vi "MarvinTester.vi"() -> ()   [LabVIEW 2017]
uses:
  <vilib>/Instr/_visa.llb/VISA Configure Serial Port (Instr).vi
panel:
  out "TX":string
  out "RX":string
  out "(hi.lo)":u32 format="%.0x"
  in  "GetOUTIO3":bool
  out "S2 GIO 19":bool
  out "S2 GIO 18":bool
  out "S2 GIO 17":bool
  out "S2 GIO 11":bool
  out "S2 GIO 3":bool
  out "S2 GIO 1":bool
  out "S1 GIO 19":bool
  out "S1 GIO 18":bool
  out "S1 GIO 17":bool
  out "S1 GIO 15":bool
  out "S1 GIO 11":bool
  out "S1 GIO 3":bool
  out "S1 GIO 1":bool
  in  "GetIO 2":bool
  out "S2 GIO 15 R":bool
  in  "Reset":bool
  in  "SetDefault":bool
  out "GetIO":u8[](array[numeric])
  out "Ver":string=" "
  in  "Get  ver":bool
  out "PWM Reading":u32
  out "Time Plot":i32=-1
  out "error out":errorcluster
  in  "stop":bool
  in  "Ring":u16(ring) items=["None", "Moment", "Get IO"]
  out "packet PWM":u8[](array[numeric])
  in  "Tab Control":enum32{"Page 3", "Page 4", "Page 2"}(tab)
  in  "GetIO2":bool
  out "out_io1":u32 format="%.0b"
  in  "SetDAC":bool
  in  "I_O":u32 format="%.0b"
  in  "ADC":bool
  in  "ADC num":u8=3
  out "out_io1 2":u32
  in  "DAC":u32
  in  "idx":i32
  in  "TA[idx]":bool
  in  "Disconect 2":bool
  in  "110":bool
  in  "120":bool
  in  "90":bool
  in  "60":bool
  in  "100":bool
  in  "20":bool
  in  "70":bool
  in  "40":bool
  in  "30":bool
  in  "80":bool
  in  "50":bool
  in  "10":bool
  in  "25":bool
  in  "0":bool
  in  "COM Port Marvin":refnum<visa-resource-name>="COM1"
  in  "Connect Marvin":bool
  out "CommIcon Marvin":bool=TRUE
  out "String":string
  in  "K15":bool
  in  "Firmeware":bool
  in  "K16":bool
  in  "K17":bool
  in  "Power":bool
  in  "Fan":bool
  in  "VEnable":bool
  out "CurrSp Graph":cluster{"n":dbl, "T":dbl}[](graph)
  out "Frequency":dbl
  in  "Plot On":bool
  in  "Plot OFF":bool
  in  "Get":bool
  in  "Clear":bool
  in  "Plot Time":i32=70
  out "Load":dbl
  out "String 2":string
  in  "COM Port Control":refnum<visa-resource-name>="COM1"
  in  "Time":i32=-1
  out "err tx":errorcluster
  out "Write array":u8[](array[numeric]) format="%x"
  in  "Flag Stop T":bool
  out "VISA":refnum<visa-resource-name>
  out "CommIcon":bool=TRUE
  out "Read array":u8[](array[numeric]) format="%x"
  out "Cmd Id":u8
  in  "Flag Stop I":bool=TRUE
  out "Int b":i32
  in  "Flag Stop R":bool
  out "TX":bool
  out "RX":bool
  in  "Command Menu 2":u16(ring) items=["Status", "Moment", "Isc threshold", "Vin Vout", "RESET FF", "Open", "Close", "Up Time", "Interval Period", "Nm Of Retries", "On time", "Save Parameters", "Version", "Temperature"]
  out "packet":u8[](array[numeric])
  in  "Isc1":i8
  in  "Add Unit":u8
  in  "Disconect":bool
  in  "Connect":bool
  in  "Stop VI":bool
  out "status":bool
  # "Marvin Tester"
  # "[Hz]"
  # "SW Version"
  # "ver : 00.01.b"
  # "I/O"
  # "ADC"
  # "DAC"
  # "0-4"
  # "V=ADC*3.3/4096"
  # "Term1  -0\nTerm2  -1\nCurr   - 2\nEBAYFAN -3\nTempCPU -4"
  # "b0-Rly1\nb1-Rly2\nb2-Rly3\n....\nb20-Rly20\nb21-Power"
  # "[kHz]"
  # "[N.m]"
  # "[msec]"
  # "ver 0.0.1"
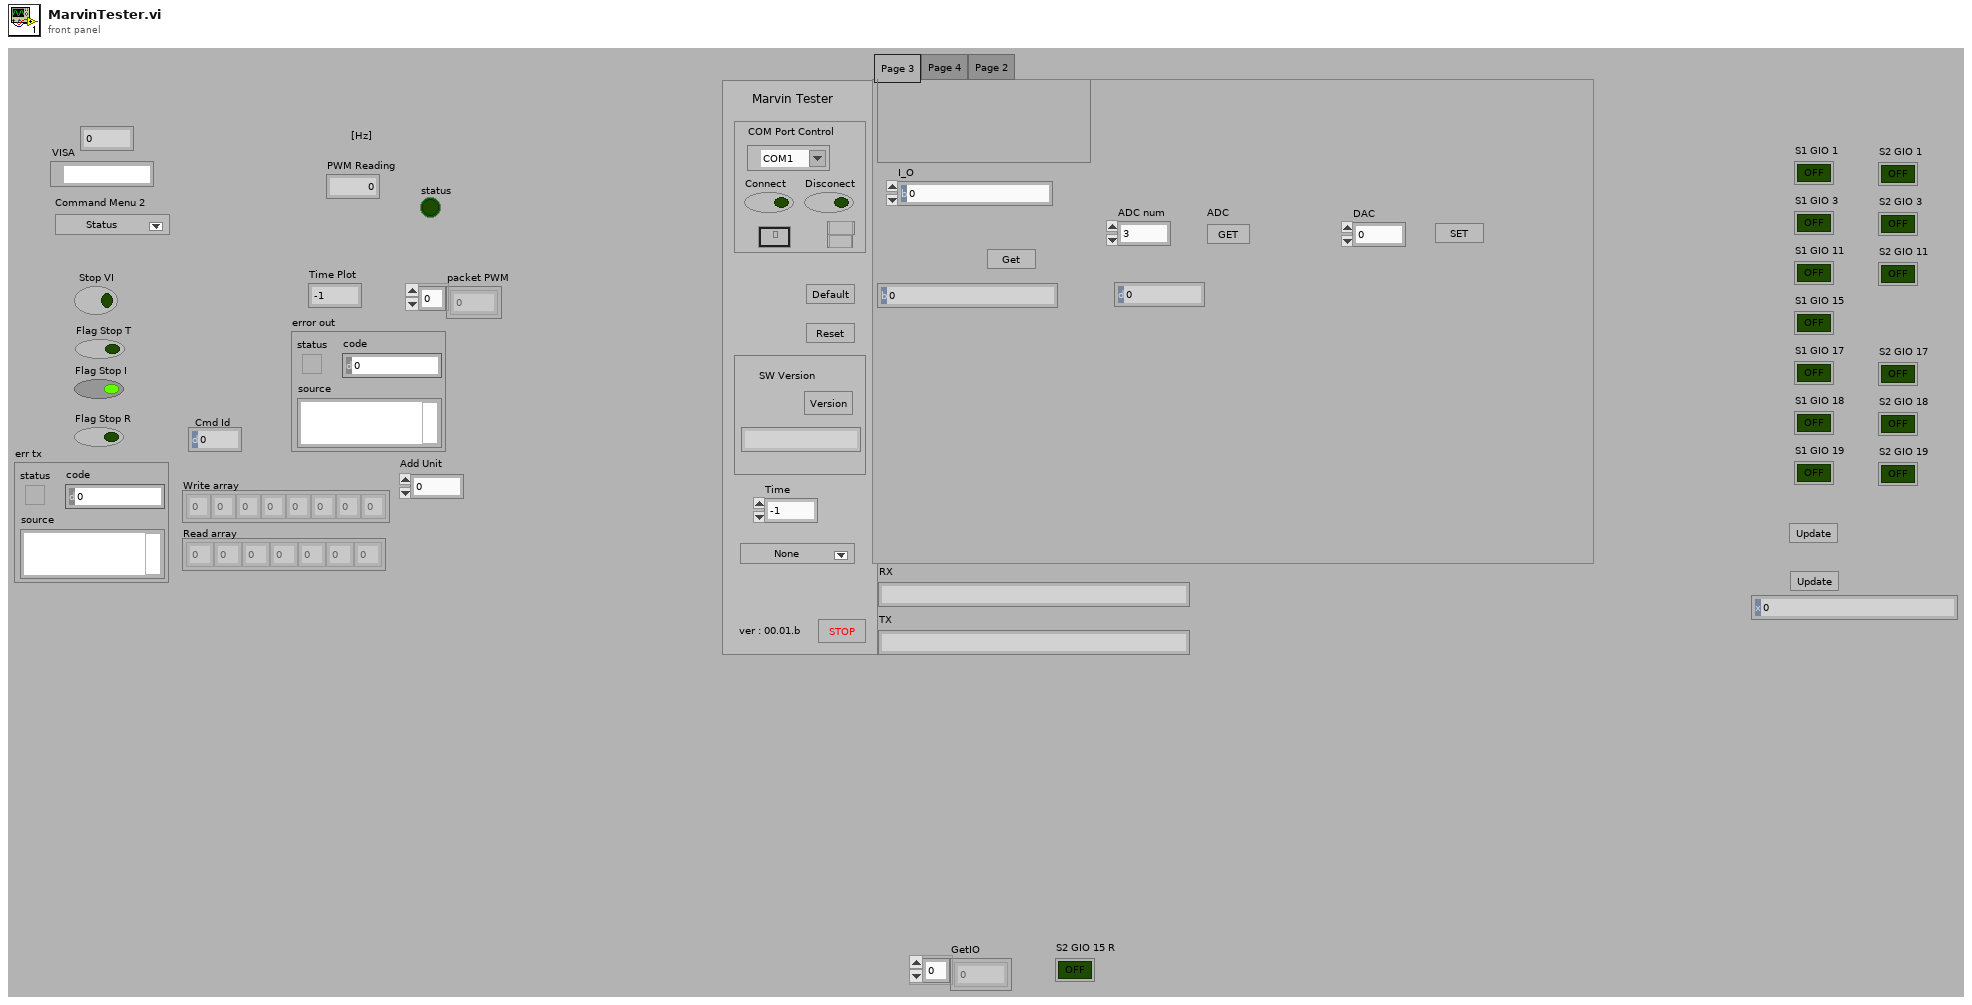
[diagram p1: front panel]
types:
  T1 = cluster{"d1":dbl, "d2":dbl, "d3":dbl, "id":u16, "d4":dbl}
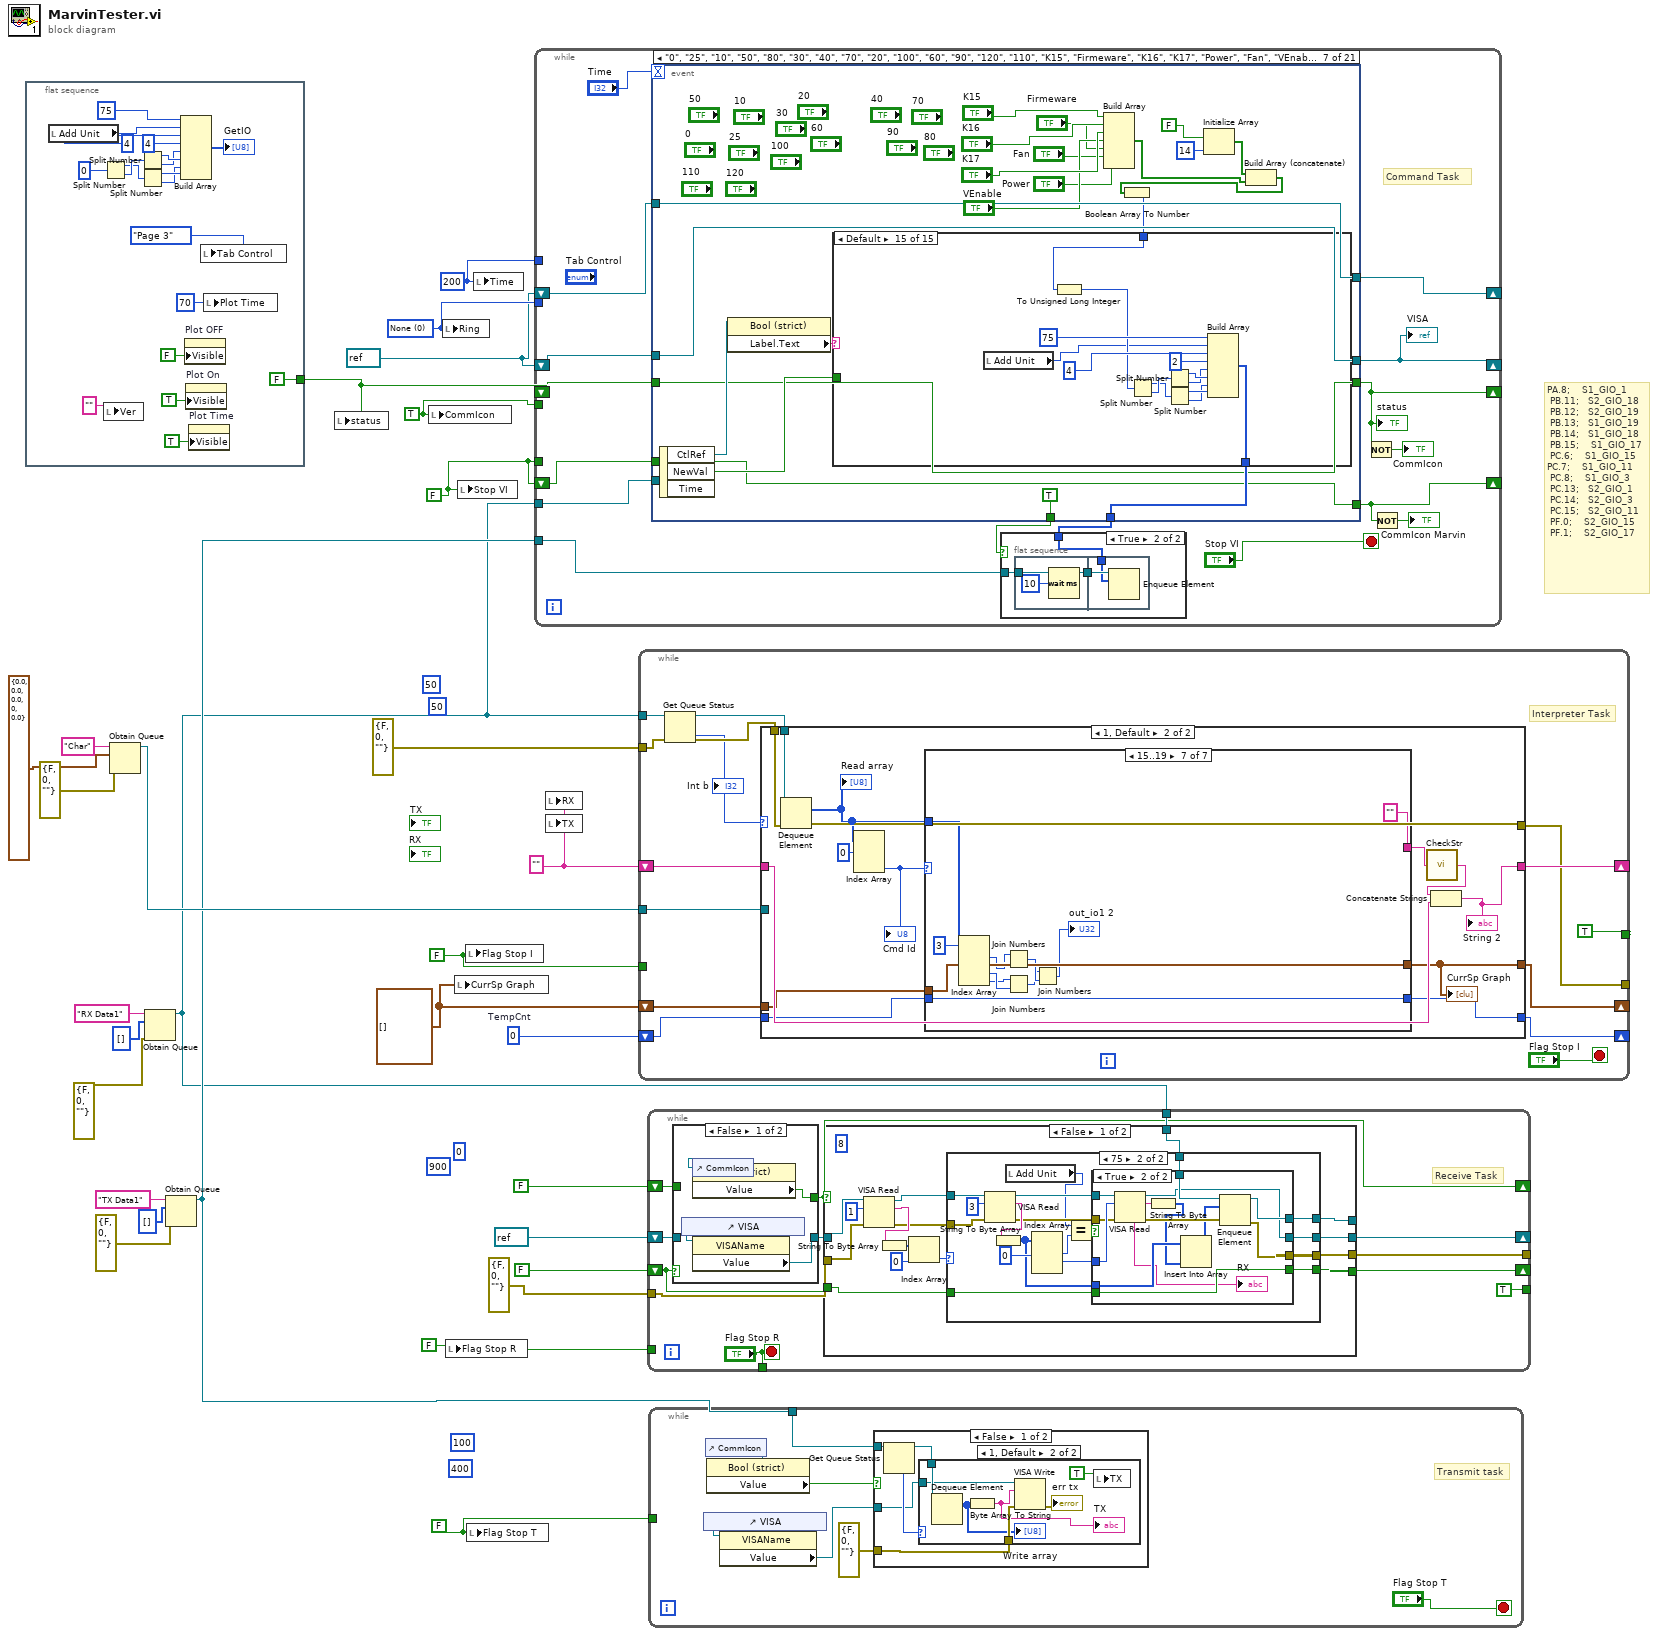
[diagram p0: block diagram]
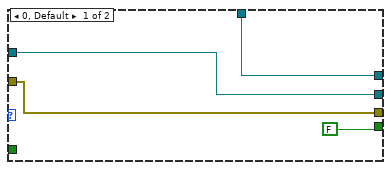
[diagram p3: hidden frame]
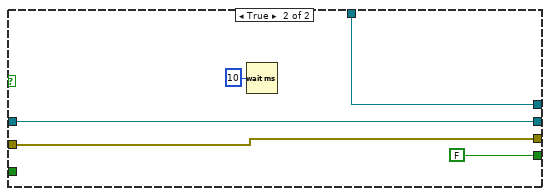
[diagram p5: hidden frame]
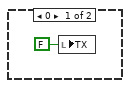
[diagram p6: hidden frame]
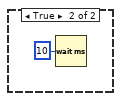
[diagram p7: hidden frame]
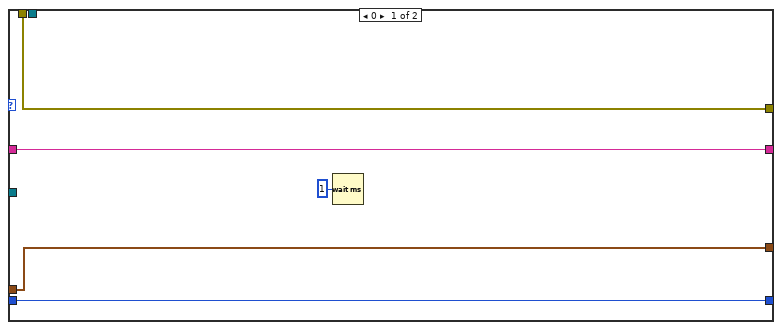
[diagram p8: hidden frame]
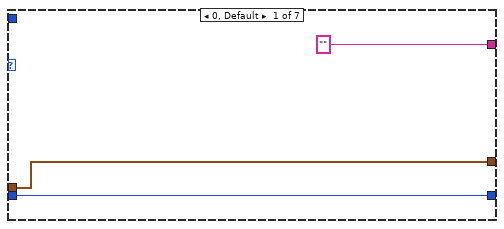
[diagram p9: hidden frame]
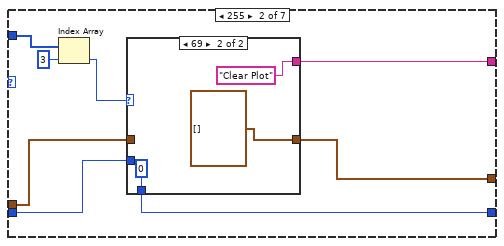
[diagram p10: hidden frame]
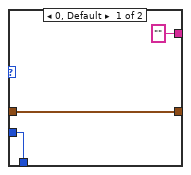
[diagram p11: hidden frame]
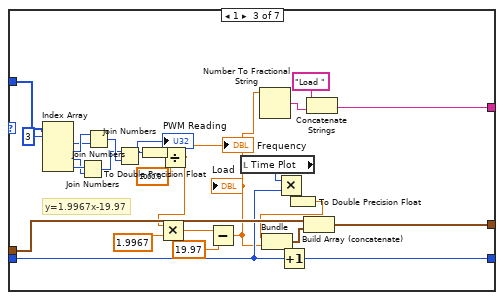
[diagram p12: hidden frame]
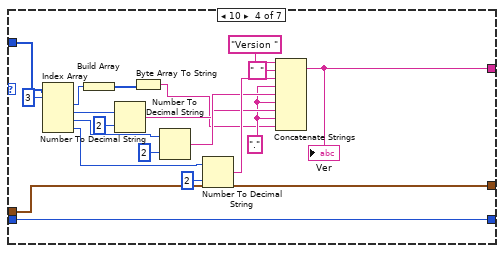
[diagram p13: hidden frame]
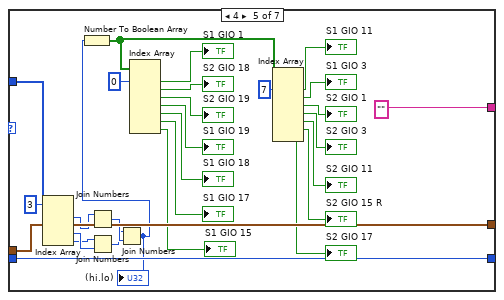
[diagram p14: hidden frame]
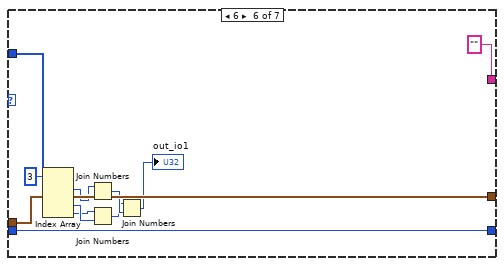
[diagram p15: hidden frame]
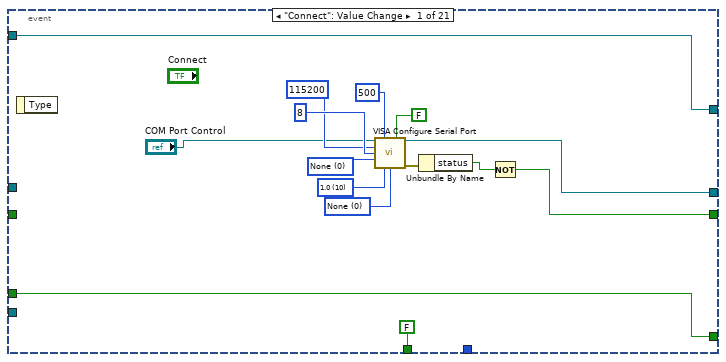
[diagram p17: hidden frame]
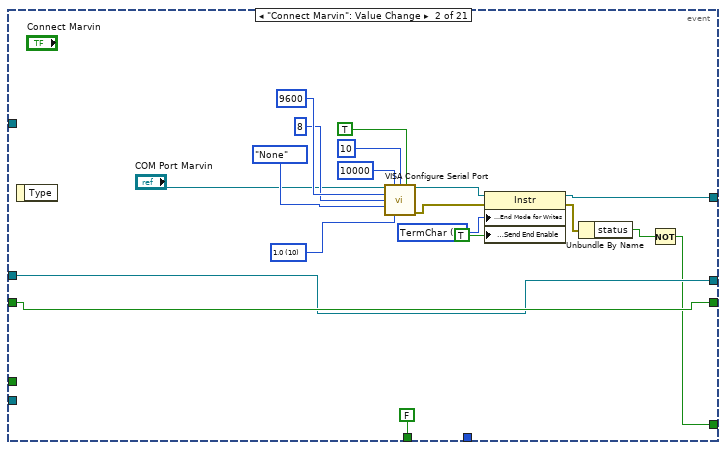
[diagram p18: hidden frame]
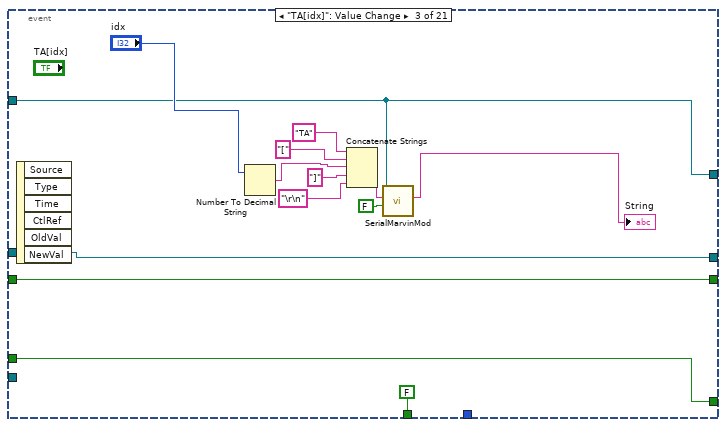
[diagram p19: hidden frame]
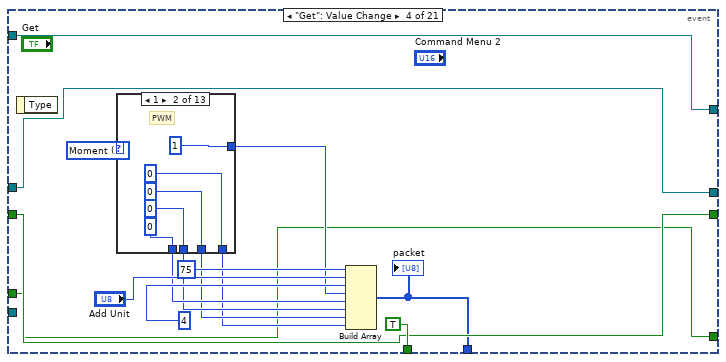
[diagram p20: hidden frame]
diagram:
  w8 = u16 0  # TempCnt
  w5 = cluster{"n":dbl, "T":dbl}[] [] ("Current Graph 4")
  w9 = 200 ("Time")
  w10 = u16 0 items=["None", "Moment"] ("Ring")
  w11 = TRUE ("CommIcon")
  w2 = FALSE
  (unwired) 400 ("Priority")
  (unwired) i64 100 ("Period")
  (unwired) i64 50 ("Period")
  (unwired) 50 ("Priority")
  (unwired) 900 ("Priority")
  (unwired) i64 0 ("Period")
  w14 = FALSE
  w1 = ""
  w28 = FALSE
  w29 = FALSE
  w3 = refnum<visa-resource-name> refnum ("VISA resource name out")
  # "PA.8;   \tS1_GIO_1\n\tPB.11;  \tS2_GIO_18\n\tPB.12;  \tS2_GIO_19\n\tPB.13;  \tS1_GIO_19\n\tPB.14;  \tS1_GIO_18\n\tPB.15;   \tS1_GIO_17\n\tPC.6;   \tS1_GIO_15\nPC.7;   \tS1_GIO_11\n\tPC.8;   \tS1_GIO_3\n\tPC.13;  \tS2_GIO_1\n\tPC.14;  \tS2_GIO_3\n\tPC.15;  \tS2_GIO_11\n\tPF.0;  \t\tS2_GIO_15\n\tPF.1;  \t\tS2_GIO_17"
  n1 = flat-sequence {
    tunnel: [FALSE] -> w7
    frame #0 {
      n2 = local read "Add Unit"() -> (w39:u8)
      n3 = Split Number(x=u32 0) -> (hi(x)=w37:u16, lo(x)=w38:u16)
      n4 = local write "Ver"("" ("Ver")) -> ()
      n5 = Split Number(x=w38) -> (hi(x)=w36:u8, lo(x)=w35:u8)
      n6 = Split Number(x=w37) -> (hi(x)=w34:u8, lo(x)=w33:u8)
      n7 = Build Array(u8 75, w39, u8 4 ("Length"), u8 4, w35, w36, w33, w34) -> (→"GetIO":u8[])
      n8 = property on="Plot OFF" class="Bool"("Visible"=FALSE) -> ()  [unwired: 2 in, 2 out]
      n9 = property on="Plot On" class="Bool"("Visible"=TRUE) -> ()  [unwired: 2 in, 2 out]
      n10 = property on="Plot Time" class="DigNum (strict)"("Visible"=TRUE) -> ()  [unwired: 2 in, 2 out]
      n11 = local write "Tab Control"(enum32{"Page 3", "Page 4", "Page 2"}."Page 3" ("Tab Control")) -> ()
      n12 = local write "Plot Time"(70 ("Plot Time")) -> ()
    }
  }
  n13 = Obtain Queue(name (unnamed)="Char", element data type=T1 {"d1"=0.0, "d2"=0.0, "d3"=0.0, "id"=0, "d4"=0.0}, error in (no error)=errorcluster {"status"=FALSE, "code"=0, "source"=""}) -> (queue out=w19:refnum<queue>)  [unwired: 2 in, 2 out]
  n14 = Obtain Queue(name (unnamed)="RX Data1", element data type=u8[] [], error in (no error)=errorcluster {"status"=FALSE, "code"=0, "source"=""}) -> (queue out=w6:refnum<queue>)  [unwired: 2 in, 2 out]
  n15 = Obtain Queue(name (unnamed)="TX Data1", element data type=u8[] [], error in (no error)=errorcluster {"status"=FALSE, "code"=0, "source"=""}) -> (queue out=w13:refnum<queue>)  [unwired: 2 in, 2 out]
  n16 = local write "status"(w7) -> ()
  n17 = local write "CommIcon"(w11) -> ()
  n18 = local write "Ring"(w10) -> ()
  n19 = local write "Flag Stop R"(w29) -> ()
  n20 = local write "CurrSp Graph"(w5) -> ()
  n21 = local write "Stop VI"(w2) -> ()
  n22 = local write "Flag Stop I"(w28) -> ()
  n23 = local write "Flag Stop T"(w14) -> ()
  n24 = local write "Time"(w9) -> ()
  n25 = while {
    shift-right: [w57] -> _
    shift-left: w3 -> [w64]
    shift-right: [w56] -> _
    shift-left: w7 -> [w63]
    tunnel: w13 -> [w59]
    tunnel: w2 -> [_]
    tunnel: w11 -> [_]
    tunnel: w10 -> [_]
    tunnel: w9 -> [_]
    tunnel: w6 -> [w54]
    shift-right: [w52] -> _
    shift-left: w3 -> [w51]
    shift-right: [w50] -> _
    shift-left: w2 -> [w49]
    stop <- "Stop VI" stop-if-true
    # "Command Task"
    n26 = event shown="[6] \"0\", \"25\", \"10\", \"50\", \"80\", \"30\", \"40\", \"70\", \"20\", \"100\", \"60\", \"90\", \"120\", \"110\", \"K15\", \"Firmeware\", \"K16\", \"K17\", \"Power\", \"Fan\", \"VEnable\": Value Change" {
      selector: _ -> [_ _ _ _ _ _ _ _ _ _ _ _ _ _ _ _ _ _ _ _ _]
      dyn-events: _ -> [_ _ _ _ _ _ _ _ _ _ _ _ _ _ _ _ _ _ _ _ _]
      timeout: "Time" -> [_ _ _ _ _ _ _ _ _ _ _ _ _ _ _ _ _ _ _ _ _]
      tunnel: [w80 w103 w109 w124 w206 w284 w315 w568 w579 w596 w613 w630 w647 w664 w693 w703 w710 w714 refnum<visa-resource-name> refnum ("VISA resource name out") w729 w738] -> w57
      tunnel: w64 -> [_ w103 w109 w124 w206 w284 w315 w568 w579 w596 w613 w630 w647 w664 w693 w703 w710 w714 w725 w729 w738]
      tunnel: [w78 w104 w108 w123 w205 w294 w314 w571 w587 w604 w621 w638 w655 w672 w695 w705 w712 FALSE FALSE w727 w737] -> w56
      tunnel: w63 -> [_ w104 w108 w123 w205 w294 w314 w571 w587 w604 w621 w638 w655 w672 w695 w705 w712 _ _ w727 w737]
      tunnel: [_ _ _ w122 w204 w293 w317 w570 w577 w594 w611 w628 w645 w662 _ _ _ _ _ _ w735] -> w58
      tunnel: [FALSE FALSE FALSE TRUE TRUE TRUE TRUE TRUE TRUE TRUE TRUE TRUE TRUE TRUE FALSE FALSE FALSE FALSE FALSE FALSE w736] -> w60
      tunnel: w54 -> [_ _ _ _ _ _ _ _ _ _ _ _ _ _ _ _ w709 _ _ _ _]
      tunnel: [w73 w90 w110 w121 w201 w282 w313 w563 w576 w593 w610 w627 w644 w661 w678 w697 w707 w715 w721 refnum<visa-resource-name> refnum ("VISA resource name out") w733] -> w52
      tunnel: w51 -> [w73 _ w110 w121 w201 w282 w313 w563 w576 w593 w610 w627 w644 w661 w678 w697 w707 w715 w721 w728 w733]
      tunnel: [w72 w87 w106 w120 w200 w281 w312 w562 w575 w592 w609 w626 w643 w660 w677 w696 w706 w713 w720 FALSE w732] -> w50
      tunnel: w49 -> [w72 _ w106 w120 w200 w281 w312 w562 w575 w592 w609 w626 w643 w660 w677 w696 w706 w713 w720 _ w732]
      event "Connect": Value Change {
        w86 = u16 0 items=["None"=0, "XON/XOFF"=1, "RTS/CTS"=2, "DTR/DSR"=4] ("flow control")
        w85 = u16 10 items=["1.0"=10, "1.5"=15, "2.0"=20] ("stop bits")
        w84 = u16 0 items=["None", "Odd", "Even", "Mark", "Space"] ("parity")
        n27 = event-data() -> ()  [unwired: 1 in, 1 out]
        n28 = call-poly "VISA Configure Serial Port"("VISA resource name"="COM Port Control", "timeout (10sec)"=u32 500, "Enable Termination\nChar (T)"=FALSE ("Enable Termination\nChar (T)"), "baud rate (9600)"=u32 115200 ("baud rate"), "data bits (8)"=u16 8 ("data bits"), "parity (0:none)"=w84, "stop bits (10: 1 bit)"=w85, "flow control (0:none)"=w86) -> ("VISA resource name out"=w80:refnum<visa-resource-name>, "error out"=w77:errorcluster)  [unwired: 6 in]
        n29 = Unbundle By Name(w77) -> ("status"=w79:bool)
        n30 = Not(x=w79) -> (.not. x?=w78:bool)
      }
      event "Connect Marvin": Value Change {
        w102 = u16 2 items=["None", "LastBit", "TermChar", "Break"] ("Serial Settings:Serial End Mode for Writes")
        w95 = u16 10 items=["1.0"=10, "1.5"=15, "2.0"=20] ("stop bits (10: 1 bit)")
        n31 = event-data() -> ()  [unwired: 1 in, 1 out]
        n32 = call-poly "VISA Configure Serial Port"("VISA resource name"="COM Port Marvin", "timeout (10sec)"=u32 10000, "termination char\n(0xA = '\\n' = LF)"=u8 10 ("termination char\n(0xA = '\\n' = LF)"), "Enable Termination\nChar (T)"=TRUE ("Enable Termination\nChar (T)"), "baud rate (9600)"=u32 9600, "data bits (8)"=u16 8, "parity (0:none)"=enum16{"None", "Odd", "Even", "Mark", "Space"}."None", "stop bits (10: 1 bit)"=w95) -> ("VISA resource name out"=w93:refnum<visa-resource-name>, "error out"=w92:errorcluster)  [unwired: 6 in]
        n33 = property class="Instr"(reference=w93, error in=w92, "Serial Settings:End Mode for Writes"=w102, "Message Based Settings:Send End Enable"=TRUE) -> (reference out=w90:refnum<visa-resource-name>, error out=w88:errorcluster)
        n34 = Unbundle By Name(w88) -> ("status"=w89:bool)
        n35 = Not(x=w89) -> (.not. x?=w87:bool)
      }
      event "TA[idx]": Value Change {
        n36 = event-data() -> ()  [unwired: 1 in, 6 out]
        n37 = Number To Decimal String(number="idx") -> (decimal integer string=w113:string)  [unwired: 1 in]
        n38 = Concatenate Strings("TA" ("string"), "[", w113, "]", "\r\n" ("write buffer")) -> (w114:string)
        n39 = call "SerialMarvinMod.vi"("Clear Log"=FALSE, "write buffer"=w114, "VISA resource name"=w110) -> ("read buffer"=→"String":string)  [unwired: 7 in, 1 out]
      }
      event "Get": Value Change {
        w126 = u16 1 items=["Status", "Moment", "Isc threshold", "Vin Vout", "RESET FF", "Open", "Close", "Up Time", "Interval Period", "Nm Of Retries", "On time", "Save Parameters", "Version", "Temperature"] ("Command Menu 3")
        n40 = event-data() -> ()  [unwired: 1 in, 1 out]
        n41 = case shown="1" w126 {
          tunnel: [u8 0 u8 1 u8 2 u8 15 u8 4 u8 4 u8 5 u8 6 u8 7 u8 8 u8 9 u8 10 u8 16] -> w131
          tunnel: [u8 0 u8 0 u8 0 u8 0 u8 0 u8 0 u8 0 u8 0 u8 0 u8 0 u8 0 u8 0 u8 0] -> w129
          tunnel: [u8 0 u8 0 u8 0 u8 0 u8 0 u8 0 u8 0 u8 0 u8 0 u8 0 u8 0 u8 0 u8 0] -> w128
          tunnel: [u8 0 u8 0 "Isc1" u8 0 u8 1 u8 0 u8 0 u8 0 u8 0 u8 0 u8 0 u8 0 u8 0] -> w130
          tunnel: [u8 0 u8 0 u8 0 u8 0 u8 0 u8 0 u8 0 u8 0 u8 0 u8 0 u8 0 u8 0 u8 0] -> w127
          frame 0, Default {
            # "Status"
          }
          frame 1 {
            # "PWM"
          }
          frame 2 {
          }
          frame 3 {
            # "Vout"
          }
          frame 5 {
          }
          frame 6 {
          }
          frame 7 {
          }
          frame 8 {
          }
          frame 9 {
          }
          frame 10 {
          }
          frame 11 {
          }
          frame 12 {
          }
          frame 13 {
          }
        }
        n42 = Build Array(u8 75, "Add Unit", u8 4 ("Length"), w131, w130, w129, w128, w127) -> (w122:u8[])
        "packet" <- w122
      }
      event "Get  ver": Value Change {
        w208 = u16 12 items=["Status", "Moment", "Isc threshold", "Vin Vout", "RESET FF", "Open", "Close", "Up Time", "Interval Period", "Nm Of Retries", "On time", "Save Parameters", "Version", "Temperature"] ("Command Menu 3")
        n43 = event-data() -> ()  [unwired: 1 in, 1 out]
        n44 = local read "Add Unit"() -> (w203:u8)
        n45 = case shown="0, Default" w208 {
          tunnel: [u8 0 u8 1 u8 2 u8 15 u8 4 u8 4 u8 5 u8 6 u8 7 u8 8 u8 9 u8 10 u8 16] -> w213
          tunnel: [u8 0 u8 0 u8 0 u8 0 u8 0 u8 0 u8 0 u8 0 u8 0 u8 0 u8 0 u8 0 u8 0] -> w211
          tunnel: [u8 0 u8 0 u8 0 u8 0 u8 0 u8 0 u8 0 u8 0 u8 0 u8 0 u8 0 u8 0 u8 0] -> w210
          tunnel: [u8 0 u8 0 u8 0 u8 0 u8 1 u8 0 u8 0 u8 0 u8 0 u8 0 u8 0 u8 0 u8 0] -> w212
          tunnel: [u8 0 u8 0 u8 0 u8 0 u8 0 u8 0 u8 0 u8 0 u8 0 u8 0 u8 0 u8 0 u8 0] -> w209
          frame 0, Default {
            # "Status"
          }
          frame 1 {
            # "PWM"
          }
          frame 2 {
          }
          frame 3 {
            # "Vout"
          }
          frame 5 {
          }
          frame 6 {
          }
          frame 7 {
          }
          frame 8 {
          }
          frame 9 {
          }
          frame 10 {
          }
          frame 11 {
          }
          frame 12 {
          }
          frame 13 {
          }
        }
        n46 = local write "Ver"("" ("Ver")) -> ()
        n47 = Build Array(u8 75, w203, u8 4 ("Length"), w213, w212, w211, w210, w209) -> (w204:u8[])
      }
      event "I_O": Value Change {
        n48 = event-data() -> ()  [unwired: 1 in, 3 out]
        n49 = local read "Add Unit"() -> (w292:u8)
        n50 = To Unsigned Long Integer(number="I_O") -> (unsigned 32bit integer=w285:u32)
        n51 = Split Number(x=w285) -> (hi(x)=w290:u16, lo(x)=w291:u16)
        n52 = Split Number(x=w291) -> (hi(x)=w289:u8, lo(x)=w288:u8)
        n53 = Split Number(x=w290) -> (hi(x)=w287:u8, lo(x)=w286:u8)
        n54 = Build Array(u8 75, w292, u8 4 ("Length"), u8 2, w288, w289, w286, w287) -> (w293:u8[])
      }
      event "0", "25", "10", "50", "80", "30", "40", "70", "20", "100", "60", "90", "120", "110", "K15", "Firmeware", "K16", "K17", "Power", "Fan", "VEnable": Value Change {
        n55 = event-data() -> ("CtlRef"=w320:refnum<vi>, "NewVal"=w318:bool)  [unwired: 1 in, 1 out]
        n56 = property class="Bool (strict)"(reference=w320) -> ("Label.Text"=w319:string)  [unwired: 1 in, 2 out]
        n57 = Build Array("K15", "K16", "K17", "VEnable", "Firmeware", "Fan", "Power") -> (w300:bool[])
        n58 = Initialize Array(FALSE, 14 ("dimension size")) -> (w301:bool[])
        n59 = Build Array (concatenate)(w301, w300) -> (w299:bool[])
        n60 = Boolean Array To Number(Boolean array=w299) -> (number=w304:u32)
        n61 = case shown="Default" w319 {
          tunnel: w318 -> [w325 w341 w356 w372 w388 w404 w420 w436 w455 w470 w489 w504 w520 w536 _]
          tunnel: [w322 w338 w353 w369 w385 w401 w417 w433 w452 w467 w486 w501 w517 w533 w549] -> w317
          tunnel: w304 -> [_ _ _ _ _ _ _ _ w451 _ w484 _ _ _ w550]
          frame "0" {
            n62 = Select(t=u32 1 ("number"), s=w325, f=u32 0) -> (s? t:f=w323:u32)
            n63 = local read "Add Unit"() -> (w326:u8)
            n64 = To Unsigned Long Integer(number=w323) -> (unsigned 32bit integer=w327:u32)
            n65 = Split Number(x=w327) -> (hi(x)=w332:u16, lo(x)=w333:u16)
            n66 = Split Number(x=w333) -> (hi(x)=w331:u8, lo(x)=w330:u8)
            n67 = Split Number(x=w332) -> (hi(x)=w329:u8, lo(x)=w328:u8)
            n68 = Build Array(u8 75, w326, u8 4 ("Length"), u8 2, w330, w331, w328, w329) -> (w322:u8[])
          }
          frame "10" {
            n69 = Select(t=u32 2 ("number"), s=w341, f=u32 0) -> (s? t:f=w339:u32)
            n70 = local read "Add Unit"() -> (w342:u8)
            n71 = To Unsigned Long Integer(number=w339) -> (unsigned 32bit integer=w343:u32)
            n72 = Split Number(x=w343) -> (hi(x)=w348:u16, lo(x)=w349:u16)
            n73 = Split Number(x=w349) -> (hi(x)=w347:u8, lo(x)=w346:u8)
            n74 = Split Number(x=w348) -> (hi(x)=w345:u8, lo(x)=w344:u8)
            n75 = Build Array(u8 75, w342, u8 4 ("Length"), u8 2, w346, w347, w344, w345) -> (w338:u8[])
          }
          frame "20" {
            n76 = Select(t=u32 4 ("number"), s=w356, f=u32 0) -> (s? t:f=w354:u32)
            n77 = local read "Add Unit"() -> (w358:u8)
            n78 = To Unsigned Long Integer(number=w354) -> (unsigned 32bit integer=w359:u32)
            n79 = Split Number(x=w359) -> (hi(x)=w364:u16, lo(x)=w365:u16)
            n80 = Split Number(x=w365) -> (hi(x)=w363:u8, lo(x)=w362:u8)
            n81 = Split Number(x=w364) -> (hi(x)=w361:u8, lo(x)=w360:u8)
            n82 = Build Array(u8 75, w358, u8 4 ("Length"), u8 2, w362, w363, w360, w361) -> (w353:u8[])
          }
          frame "25" {
            n83 = Select(t=u32 8 ("number"), s=w372, f=u32 0) -> (s? t:f=w370:u32)
            n84 = local read "Add Unit"() -> (w374:u8)
            n85 = To Unsigned Long Integer(number=w370) -> (unsigned 32bit integer=w375:u32)
            n86 = Split Number(x=w375) -> (hi(x)=w380:u16, lo(x)=w381:u16)
            n87 = Split Number(x=w381) -> (hi(x)=w379:u8, lo(x)=w378:u8)
            n88 = Split Number(x=w380) -> (hi(x)=w377:u8, lo(x)=w376:u8)
            n89 = Build Array(u8 75, w374, u8 4 ("Length"), u8 2, w378, w379, w376, w377) -> (w369:u8[])
          }
          frame "30" {
            n90 = Select(t=u32 16 ("number"), s=w388, f=u32 0) -> (s? t:f=w386:u32)
            n91 = local read "Add Unit"() -> (w390:u8)
            n92 = To Unsigned Long Integer(number=w386) -> (unsigned 32bit integer=w391:u32)
            n93 = Split Number(x=w391) -> (hi(x)=w396:u16, lo(x)=w397:u16)
            n94 = Split Number(x=w397) -> (hi(x)=w395:u8, lo(x)=w394:u8)
            n95 = Split Number(x=w396) -> (hi(x)=w393:u8, lo(x)=w392:u8)
            n96 = Build Array(u8 75, w390, u8 4 ("Length"), u8 2, w394, w395, w392, w393) -> (w385:u8[])
          }
          frame "40" {
            n97 = Select(t=u32 32 ("number"), s=w404, f=u32 0) -> (s? t:f=w402:u32)
            n98 = local read "Add Unit"() -> (w406:u8)
            n99 = To Unsigned Long Integer(number=w402) -> (unsigned 32bit integer=w407:u32)
            n100 = Split Number(x=w407) -> (hi(x)=w412:u16, lo(x)=w413:u16)
            n101 = Split Number(x=w413) -> (hi(x)=w411:u8, lo(x)=w410:u8)
            n102 = Split Number(x=w412) -> (hi(x)=w409:u8, lo(x)=w408:u8)
            n103 = Build Array(u8 75, w406, u8 4 ("Length"), u8 2, w410, w411, w408, w409) -> (w401:u8[])
          }
          frame "50" {
            n104 = Select(t=u32 64 ("number"), s=w420, f=u32 0) -> (s? t:f=w418:u32)
            n105 = local read "Add Unit"() -> (w422:u8)
            n106 = To Unsigned Long Integer(number=w418) -> (unsigned 32bit integer=w423:u32)
            n107 = Split Number(x=w423) -> (hi(x)=w428:u16, lo(x)=w429:u16)
            n108 = Split Number(x=w429) -> (hi(x)=w427:u8, lo(x)=w426:u8)
            n109 = Split Number(x=w428) -> (hi(x)=w425:u8, lo(x)=w424:u8)
            n110 = Build Array(u8 75, w422, u8 4 ("Length"), u8 2, w426, w427, w424, w425) -> (w417:u8[])
          }
          frame "60" {
            n111 = Select(t=u32 128 ("number"), s=w436, f=u32 0) -> (s? t:f=w434:u32)
            n112 = local read "Add Unit"() -> (w438:u8)
            n113 = To Unsigned Long Integer(number=w434) -> (unsigned 32bit integer=w439:u32)
            n114 = Split Number(x=w439) -> (hi(x)=w444:u16, lo(x)=w445:u16)
            n115 = Split Number(x=w445) -> (hi(x)=w443:u8, lo(x)=w442:u8)
            n116 = Split Number(x=w444) -> (hi(x)=w441:u8, lo(x)=w440:u8)
            n117 = Build Array(u8 75, w438, u8 4 ("Length"), u8 2, w442, w443, w440, w441) -> (w433:u8[])
          }
          frame "70" {
            n118 = Select(t=u32 256 ("number"), s=w455, f=u32 0) -> (s? t:f=w453:u32)
            n119 = local read "Add Unit"() -> (w457:u8)
            n120 = To Unsigned Long Integer(number=w453) -> (unsigned 32bit integer=w450:u32)
            n121 = Or(x=w451, y=w450) -> (x .or. y?=w449:u32)
            n122 = Split Number(x=w449) -> (hi(x)=w462:u16, lo(x)=w463:u16)
            n123 = Split Number(x=w463) -> (hi(x)=w461:u8, lo(x)=w460:u8)
            n124 = Split Number(x=w462) -> (hi(x)=w459:u8, lo(x)=w458:u8)
            n125 = Build Array(u8 75, w457, u8 4 ("Length"), u8 2, w460, w461, w458, w459) -> (w452:u8[])
          }
          frame "80" {
            n126 = Select(t=u32 512 ("number"), s=w470, f=u32 0) -> (s? t:f=w468:u32)
            n127 = local read "Add Unit"() -> (w472:u8)
            n128 = To Unsigned Long Integer(number=w468) -> (unsigned 32bit integer=w473:u32)
            n129 = Split Number(x=w473) -> (hi(x)=w478:u16, lo(x)=w479:u16)
            n130 = Split Number(x=w479) -> (hi(x)=w477:u8, lo(x)=w476:u8)
            n131 = Split Number(x=w478) -> (hi(x)=w475:u8, lo(x)=w474:u8)
            n132 = Build Array(u8 75, w472, u8 4 ("Length"), u8 2, w476, w477, w474, w475) -> (w467:u8[])
          }
          frame "90" {
            n133 = Select(t=u32 1024 ("number"), s=w489, f=u32 0) -> (s? t:f=w487:u32)
            n134 = local read "Add Unit"() -> (w491:u8)
            n135 = To Unsigned Long Integer(number=w487) -> (unsigned 32bit integer=w485:u32)
            n136 = Or(x=w484, y=w485) -> (x .or. y?=w483:u32)
            n137 = Split Number(x=w483) -> (hi(x)=w496:u16, lo(x)=w497:u16)
            n138 = Split Number(x=w497) -> (hi(x)=w495:u8, lo(x)=w494:u8)
            n139 = Split Number(x=w496) -> (hi(x)=w493:u8, lo(x)=w492:u8)
            n140 = Build Array(u8 75, w491, u8 4 ("Length"), u8 2, w494, w495, w492, w493) -> (w486:u8[])
          }
          frame "100" {
            n141 = Select(t=u32 2048 ("number"), s=w504, f=u32 0) -> (s? t:f=w502:u32)
            n142 = local read "Add Unit"() -> (w506:u8)
            n143 = To Unsigned Long Integer(number=w502) -> (unsigned 32bit integer=w507:u32)
            n144 = Split Number(x=w507) -> (hi(x)=w512:u16, lo(x)=w513:u16)
            n145 = Split Number(x=w513) -> (hi(x)=w511:u8, lo(x)=w510:u8)
            n146 = Split Number(x=w512) -> (hi(x)=w509:u8, lo(x)=w508:u8)
            n147 = Build Array(u8 75, w506, u8 4 ("Length"), u8 2, w510, w511, w508, w509) -> (w501:u8[])
          }
          frame "110" {
            n148 = local read "Add Unit"() -> (w522:u8)
            n149 = Select(t=u32 8192 ("number"), s=w520, f=u32 0) -> (s? t:f=w518:u32)
            n150 = To Unsigned Long Integer(number=w518) -> (unsigned 32bit integer=w523:u32)
            n151 = Split Number(x=w523) -> (hi(x)=w528:u16, lo(x)=w529:u16)
            n152 = Split Number(x=w529) -> (hi(x)=w527:u8, lo(x)=w526:u8)
            n153 = Split Number(x=w528) -> (hi(x)=w525:u8, lo(x)=w524:u8)
            n154 = Build Array(u8 75, w522, u8 4 ("Length"), u8 2, w526, w527, w524, w525) -> (w517:u8[])
          }
          frame "120" {
            n155 = Select(t=u32 4096 ("number"), s=w536, f=u32 0) -> (s? t:f=w534:u32)
            n156 = local read "Add Unit"() -> (w538:u8)
            n157 = To Unsigned Long Integer(number=w534) -> (unsigned 32bit integer=w539:u32)
            n158 = Split Number(x=w539) -> (hi(x)=w544:u16, lo(x)=w545:u16)
            n159 = Split Number(x=w545) -> (hi(x)=w543:u8, lo(x)=w542:u8)
            n160 = Split Number(x=w544) -> (hi(x)=w541:u8, lo(x)=w540:u8)
            n161 = Build Array(u8 75, w538, u8 4 ("Length"), u8 2, w542, w543, w540, w541) -> (w533:u8[])
          }
          frame Default {
            n162 = local read "Add Unit"() -> (w551:u8)
            n163 = To Unsigned Long Integer(number=w550) -> (unsigned 32bit integer=w552:u32)
            n164 = Split Number(x=w552) -> (hi(x)=w557:u16, lo(x)=w558:u16)
            n165 = Split Number(x=w558) -> (hi(x)=w556:u8, lo(x)=w555:u8)
            n166 = Split Number(x=w557) -> (hi(x)=w554:u8, lo(x)=w553:u8)
            n167 = Build Array(u8 75, w551, u8 4 ("Length"), u8 2, w555, w556, w553, w554) -> (w549:u8[])
          }
        }
      }
      event "ADC": Value Change {
        w564 = u8 0 ("element")
        n168 = event-data() -> ()  [unwired: 1 in, 3 out]
        n169 = local read "Add Unit"() -> (w569:u8)
        n170 = Add(x="ADC num", y=u8 15) -> (x+y=w566:u8)
        n171 = Build Array(u8 75, w569, u8 4 ("Length"), w566, w564, w564, w564, w564) -> (w570:u8[])
      }
      event "GetIO 2": Value Change {
        n172 = event-data() -> ()  [unwired: 1 in, 1 out]
        n173 = local read "Add Unit"() -> (w586:u8)
        n174 = Split Number(x=u32 0) -> (hi(x)=w584:u16, lo(x)=w585:u16)
        n175 = Split Number(x=w585) -> (hi(x)=w583:u8, lo(x)=w582:u8)
        n176 = Split Number(x=w584) -> (hi(x)=w581:u8, lo(x)=w580:u8)
        n177 = Build Array(u8 75, w586, u8 4 ("Length"), u8 4, w582, w583, w580, w581) -> (w577:u8[])
        n178 = local write "GetIO"(w577) -> ()
      }
      event "SetDefault": Value Change {
        n179 = event-data() -> ()  [unwired: 1 in, 1 out]
        n180 = local read "Add Unit"() -> (w603:u8)
        n181 = Split Number(x=u32 0) -> (hi(x)=w601:u16, lo(x)=w602:u16)
        n182 = Split Number(x=w602) -> (hi(x)=w600:u8, lo(x)=w599:u8)
        n183 = Split Number(x=w601) -> (hi(x)=w598:u8, lo(x)=w597:u8)
        n184 = Build Array(u8 75, w603, u8 4 ("Length"), u8 9, w599, w600, w597, w598) -> (w594:u8[])
        n185 = local write "GetIO"(w594) -> ()
      }
      event "Reset": Value Change {
        n186 = event-data() -> ()  [unwired: 1 in, 1 out]
        n187 = local read "Add Unit"() -> (w620:u8)
        n188 = Split Number(x=u32 0) -> (hi(x)=w618:u16, lo(x)=w619:u16)
        n189 = Split Number(x=w619) -> (hi(x)=w617:u8, lo(x)=w616:u8)
        n190 = Split Number(x=w618) -> (hi(x)=w615:u8, lo(x)=w614:u8)
        n191 = Build Array(u8 75, w620, u8 4 ("Length"), u8 11, w616, w617, w614, w615) -> (w611:u8[])
        n192 = local write "GetIO"(w611) -> ()
      }
      event "GetIO2": Value Change {
        n193 = event-data() -> ()  [unwired: 1 in, 1 out]
        n194 = local read "Add Unit"() -> (w637:u8)
        n195 = Split Number(x=u32 0) -> (hi(x)=w635:u16, lo(x)=w636:u16)
        n196 = Split Number(x=w636) -> (hi(x)=w634:u8, lo(x)=w633:u8)
        n197 = Split Number(x=w635) -> (hi(x)=w632:u8, lo(x)=w631:u8)
        n198 = Build Array(u8 75, w637, u8 4 ("Length"), u8 6, w633, w634, w631, w632) -> (w628:u8[])
      }
      event "SetDAC": Value Change {
        n199 = event-data() -> ()  [unwired: 1 in, 1 out]
        n200 = local read "Add Unit"() -> (w654:u8)
        n201 = Split Number(x="DAC") -> (hi(x)=w652:u16, lo(x)=w653:u16)
        n202 = Split Number(x=w653) -> (hi(x)=w651:u8, lo(x)=w650:u8)
        n203 = Split Number(x=w652) -> (hi(x)=w649:u8, lo(x)=w648:u8)
        n204 = Build Array(u8 75, w654, u8 4 ("Length"), u8 7, w650, w651, w648, w649) -> (w645:u8[])
      }
      event "GetOUTIO3": Value Change {
        n205 = event-data() -> ()  [unwired: 1 in, 1 out]
        n206 = local read "Add Unit"() -> (w671:u8)
        n207 = Split Number(x=u32 0) -> (hi(x)=w669:u16, lo(x)=w670:u16)
        n208 = Split Number(x=w670) -> (hi(x)=w668:u8, lo(x)=w667:u8)
        n209 = Split Number(x=w669) -> (hi(x)=w666:u8, lo(x)=w665:u8)
        n210 = Build Array(u8 75, w671, u8 4 ("Length"), u8 8, w667, w668, w665, w666) -> (w662:u8[])
      }
      event "Plot On": Value Change {
        w683 = u16 1 items=["None", "Moment"] ("Ring")
        n211 = event-data() -> ()  [unwired: 1 in, 1 out]
        n212 = local read "Add Unit"() -> (w692:u8)
        n213 = local write "Ring"(w683) -> ()
        n214 = Build Array(u8 75, w692, u8 4 ("Length"), u8 1, u8 0, u8 0, u8 0, u8 0) -> (→"packet PWM":u8[])
        n215 = local write "Time"("Plot Time") -> ()
        n216 = property on="Plot OFF" class="Bool"("Visible"=TRUE) -> ()  [unwired: 2 in, 2 out]
        n217 = property on="Plot On" class="Bool"("Visible"=FALSE) -> ()  [unwired: 2 in, 2 out]
        n218 = property on="Plot Time" class="DigNum (strict)"("Visible"=FALSE) -> ()  [unwired: 2 in, 2 out]
        "Time Plot" <- "Plot Time"
      }
      event "Plot OFF": Value Change {
        w702 = u16 0 items=["None", "Moment"] ("Ring")
        n219 = event-data() -> ()  [unwired: 1 in, 5 out]
        n220 = local write "Time"(200 ("Time")) -> ()
        n221 = local write "Ring"(w702) -> ()
        n222 = property on="Plot Time" class="DigNum (strict)"("Visible"=TRUE) -> ()  [unwired: 2 in, 2 out]
        n223 = property on="Plot OFF" class="Bool"("Visible"=FALSE) -> ()  [unwired: 2 in, 2 out]
        n224 = property on="Plot On" class="Bool"("Visible"=TRUE) -> ()  [unwired: 2 in, 2 out]
      }
      event "Clear": Value Change {
        n225 = event-data() -> ()  [unwired: 1 in, 5 out]
        n226 = Enqueue Element(queue=w709, element=u8[] [0, 0, 255, 69]) -> ()  [unwired: 1 in, 4 out]
      }
      event "stop": Value Change {
        w716 = TRUE ("Flag Stop R")
        n227 = event-data() -> ()  [unwired: 1 in, 5 out]
        n228 = VISA Close(VISA resource name=w714) -> (error out=→"error out":errorcluster)  [unwired: 1 in]
        n229 = local write "Flag Stop T"(w716) -> ()
        n230 = local write "Flag Stop R"(w716) -> ()
        n231 = local write "Flag Stop I"(w716) -> ()
        n232 = local write "Stop VI"(w716) -> ()
      }
      event "Disconect": Value Change {
        n233 = event-data() -> ()  [unwired: 1 in, 5 out]
        n234 = VISA Close(VISA resource name=w725) -> ()  [unwired: 1 in, 1 out]
      }
      event "Disconect 2": Value Change {
        n235 = event-data() -> ()  [unwired: 1 in, 5 out]
        n236 = VISA Close(VISA resource name=w728) -> ()  [unwired: 1 in, 1 out]
      }
      event Timeout {
        n237 = event-data() -> ()  [unwired: 1 in, 1 out]
        n238 = case shown="0, Default" "Ring" {
          tunnel: [FALSE TRUE TRUE] -> w736
          tunnel: [u8[] [] ("packet PWM") w741 w743] -> w735
          frame 0, Default {
          }
          frame 1 {
            n239 = local read "packet PWM"() -> (w741:u8[])
          }
          frame 2 {
            n240 = local read "GetIO"() -> (w743:u8[])
          }
        }
      }
    }
    "status" <- w56
    "VISA" <- w57
    n241 = case shown="True" w60 {
      tunnel: w59 -> [_ w67]
      tunnel: w58 -> [_ w66]
      frame False {
      }
      frame True {
        n242 = flat-sequence {
          tunnel: w67 -> [w69]
          tunnel: [w69] -> w65
          tunnel: w66 -> [w70]
          tunnel: w65 -> [w71]
          frame #0 {
            n243 = Wait (ms)(milliseconds to wait=u32 10) -> ()  [unwired: 1 out]
          }
          frame #1 {
            n244 = Enqueue Element(queue=w71, element=w70) -> ()  [unwired: 1 in, 4 out]
          }
        }
      }
    }
    n245 = Not(x=w56) -> (.not. x?=→"CommIcon":bool)
    n246 = Not(x=w50) -> (.not. x?=→"CommIcon Marvin":bool)
  }
  n247 = local write "RX"(w1) -> ()
  n248 = local write "TX"(w1) -> ()
  n249 = while {
    tunnel: w6 -> [w759]
    tunnel: errorcluster {"status"=FALSE, "code"=0, "source"=""} ("error out") -> [w758]
    tunnel: [w749] -> _
    tunnel: w28 -> [_]
    tunnel: [TRUE] -> _
    shift-right: [w754] -> _
    shift-left: w1 -> [w753]
    tunnel: w19 -> [w751]
    shift-right: [w745] -> _
    shift-left: w5 -> [w748]
    shift-right: [w746] -> _
    shift-left: w8 -> [w747]
    stop <- "Flag Stop I" stop-if-true
    # "Interpreter Task"
    n250 = Get Queue Status(queue=w759, error in (no error)=w758) -> (queue out=w757:refnum<queue>, error out=w752:errorcluster, # elements in queue=w750:i32)  [unwired: 6 out]
    "Int b" <- w750
    n251 = case shown="1, Default" w750 {
      tunnel: w757 -> [_ w778]
      tunnel: w752 -> [w764 w776]
      tunnel: [w764 w777] -> w749
      tunnel: [w763 w773] -> w754
      tunnel: w753 -> [w763 w775]
      tunnel: w751 -> [_ _]
      tunnel: w748 -> [w762 w768]
      tunnel: [w762 w765] -> w745
      tunnel: w747 -> [w761 w767]
      tunnel: [w761 w766] -> w746
      frame 0 {
        n252 = Wait (ms)(milliseconds to wait=u32 1) -> ()  [unwired: 1 out]
      }
      frame 1, Default {
        n253 = Dequeue Element(queue=w778, error in (no error)=w776) -> (element=w774:u8[], error out=w777:errorcluster)  [unwired: 3 out]
        "Read array" <- w774
        n254 = Index Array(array=w774, index #1=0 ("index")) -> (element #3=w770:u8)  [unwired: 2 in, 2 out]
        "Cmd Id" <- w770
        n255 = case shown="15..19" w770 {
          tunnel: w774 -> [_ w789 w814 w838 w868 w880 w892]
          tunnel: ["" w786 w813 w825 "" "" ""] -> w769
          tunnel: w768 -> [w780 w785 w808 w840 w870 w882 w894]
          tunnel: [w780 w784 w807 w840 w870 w882 w894] -> w765
          tunnel: w767 -> [w779 w783 w806 w839 w869 w881 w893]
          tunnel: [w779 w782 w803 w839 w869 w881 w893] -> w766
          frame 0, Default {
          }
          frame 255 {
            n256 = Index Array(array=w789, index=3) -> (element=w787:u8)
            n257 = case shown="69" w787 {
              tunnel: ["" "Clear Plot"] -> w786
              tunnel: [w792 cluster{"n":dbl, "T":dbl}[] [] ("Current Graph 4")] -> w784
              tunnel: w785 -> [w792 _]
              tunnel: w783 -> [w790 _]
              tunnel: [w790 u16 0 ("TempCnt")] -> w782
              frame 0, Default {
              }
              frame 69 {
              }
            }
          }
          frame 1 {
            # "y=1.9967x-19.97"
            n258 = Index Array(array=w814, index #1=3 ("index")) -> (element #1=w817:u8, element #2=w819:u8, element #3=w820:u8, element #4=w821:u8)  [unwired: 3 in]
            n259 = Join Numbers(hi=w821, lo=w820) -> ((hi.lo)=w815:u16)
            n260 = Join Numbers(hi=w819, lo=w817) -> ((hi.lo)=w816:u16)
            n261 = Join Numbers(hi=w815, lo=w816) -> ((hi.lo)=w812:u32)
            "PWM Reading" <- w812
            n262 = To Double Precision Float(number=w812) -> (double precision float=w811:dbl)
            n263 = Divide(x=w811, y=1000.0) -> (x/y=w800:dbl)
            "Frequency" <- w800
            n264 = Multiply(x=w800, y=1.9967) -> (x*y=w799:dbl)
            n265 = Subtract(x=w799, y=19.97) -> (x-y=w796:dbl)
            "Load" <- w796
            n266 = local read "Time Plot"() -> (w802:i32)
            n267 = Number To Fractional String(number=w796) -> (F-format string=w797:string)  [unwired: 3 in]
            n268 = Multiply(x=w802, y=w806) -> (x*y=w805:i32)
            n269 = Increment(x=w806) -> (x+1=w803:u16)
            n270 = To Double Precision Float(number=w805) -> (double precision float=w804:dbl)
            n271 = Bundle(w804, w796) -> (w809:cluster{dbl, dbl})  [unwired: 1 in]
            n272 = Build Array (concatenate)(w808, w809) -> (w807:cluster{"n":dbl, "T":dbl}[])
            n273 = Concatenate Strings("Load ", w797) -> (w813:string)
          }
          frame 10 {
            w824 = "." ("string")
            n274 = Index Array(array=w838, index #1=3 ("index")) -> (element #1=w834:u8, element #2=w837:u8, element #3=w836:u8, element #4=w835:u8)  [unwired: 3 in]
            n275 = Build Array(w834) -> (w833:u8[])
            n276 = Number To Decimal String(number=w837, width (-)=i16 2) -> (decimal integer string=w829:string)
            n277 = Byte Array To String(unsigned byte array=w833) -> (string=w823:string)
            n278 = Number To Decimal String(number=w836, width (-)=i16 2) -> (decimal integer string=w830:string)
            n279 = Number To Decimal String(number=w835, width (-)=i16 2) -> (decimal integer string=w832:string)
            n280 = Concatenate Strings("Version ", "  " ("string"), w832, w824, w830, w824, w829, w824, w823) -> (w825:string)
            "Ver" <- w825
          }
          frame 4 {
            n281 = Index Array(array=w868, index #1=3 ("index")) -> (element #1=w866:u8, element #2=w865:u8, element #3=w864:u8, element #4=w863:u8)  [unwired: 3 in]
            n282 = Join Numbers(hi=w865, lo=w866) -> ((hi.lo)=w862:u16)
            n283 = Join Numbers(hi=w863, lo=w864) -> ((hi.lo)=w861:u16)
            n284 = Join Numbers(hi=w861, lo=w862) -> ((hi.lo)=w860:u32)
            "(hi.lo)" <- w860
            n285 = Number To Boolean Array(number=w860) -> (Boolean array=w850:bool[])
            n286 = Index Array(array=w850, index #1=0 ("index")) -> (element #1=→"S1 GIO 1":bool, element #2=→"S2 GIO 18":bool, element #3=→"S2 GIO 19":bool, element #4=→"S1 GIO 19":bool, element #5=→"S1 GIO 18":bool, element #6=→"S1 GIO 17":bool, element #7=→"S1 GIO 15":bool)  [unwired: 6 in]
            n287 = Index Array(array=w850, index #1=7 ("index")) -> (element #1=→"S1 GIO 11":bool, element #2=→"S1 GIO 3":bool, element #3=→"S2 GIO 1":bool, element #4=→"S2 GIO 3":bool, element #5=→"S2 GIO 11":bool, element #6=→"S2 GIO 15 R":bool, element #7=→"S2 GIO 17":bool)  [unwired: 6 in]
          }
          frame 6 {
            n288 = Index Array(array=w880, index #1=3 ("index")) -> (element #1=w878:u8, element #2=w877:u8, element #3=w876:u8, element #4=w875:u8)  [unwired: 3 in]
            n289 = Join Numbers(hi=w877, lo=w878) -> ((hi.lo)=w874:u16)
            n290 = Join Numbers(hi=w875, lo=w876) -> ((hi.lo)=w873:u16)
            n291 = Join Numbers(hi=w873, lo=w874) -> ((hi.lo)=→"out_io1":u32)
          }
          frame 15..19 {
            n292 = Index Array(array=w892, index #1=3 ("index")) -> (element #1=w890:u8, element #2=w889:u8, element #3=w888:u8, element #4=w887:u8)  [unwired: 3 in]
            n293 = Join Numbers(hi=w889, lo=w890) -> ((hi.lo)=w886:u16)
            n294 = Join Numbers(hi=w887, lo=w888) -> ((hi.lo)=w885:u16)
            n295 = Join Numbers(hi=w885, lo=w886) -> ((hi.lo)=→"out_io1 2":u32)
          }
        }
        "CurrSp Graph" <- w765
        n296 = call "CheckStr.vi"("String"=w769) -> ("s? t:f"=w771:string)
        n297 = Concatenate Strings(w771, w775) -> (w773:string)
        "String 2" <- w773
      }
    }
  }
  n298 = while {
    tunnel: [TRUE] -> _
    tunnel: w29 -> [_]
    tunnel: w6 -> [w905]
    tunnel: [w904] -> _
    tunnel: errorcluster {"status"=FALSE, "code"=0, "source"=""} -> [w903]
    shift-right: [w902] -> _
    shift-left: refnum<visa-resource-name> refnum ("Value") -> [w899]
    shift-right: [w900] -> _
    shift-left: FALSE ("Value") -> [w898]
    shift-right: [w901] -> _
    shift-left: FALSE ("Plot_T") -> [w897]
    tunnel: ["Flag Stop R"] -> _
    stop <- "Flag Stop R" stop-if-true
    # "Receive Task"
    n299 = case shown="False" w897 {
      tunnel: [w911 w913] -> w907
      tunnel: [w908 w912] -> w900
      tunnel: w899 -> [_ w913]
      tunnel: w898 -> [_ w912]
      frame False {
        n300 = control-ref of="VISA"() -> (w910:refnum<vi>)
        n301 = control-ref of="CommIcon"() -> (w909:refnum<vi>)
        n302 = property class="Bool (strict)"(reference=w909) -> ("Value"=w908:bool)  [unwired: 1 in, 2 out]
        n303 = property class="VISAName"(reference=w910) -> ("Value"=w911:refnum<visa-resource-name>)  [unwired: 1 in, 2 out]
      }
      frame True {
      }
    }
    n304 = case shown="False" w900 {
      tunnel: w903 -> [w926 w971]
      tunnel: w907 -> [w923 w972]
      tunnel: [w915 w972] -> w902
      tunnel: [w927 w971] -> w904
      tunnel: w905 -> [w916 w970]
      tunnel: [w928 w970] -> _
      tunnel: [w925 FALSE ("Plot_T")] -> w901
      tunnel: w897 -> [w914 _]
      frame False {
        (unwired) u32 8 ("byte count")
        n305 = VISA Read(VISA resource name=w923, byte count=u32 1, error in (no error)=w926) -> (VISA resource name out=w918:refnum<visa-resource-name>, read buffer=w919:string, error out=w917:errorcluster)  [unwired: 1 out]
        n306 = String To Byte Array(string=w919) -> (unsigned byte array=w922:u8[])
        n307 = Index Array(array=w922, index=0) -> (element=w920:u8)
        n308 = case shown="75" w920 {
          tunnel: [w932 w950] -> w928
          tunnel: [w931 w949] -> w927
          tunnel: [FALSE w948] -> w925
          tunnel: w918 -> [w929 w944]
          tunnel: w917 -> [w931 w943]
          tunnel: w916 -> [w932 w936]
          tunnel: [w929 w935] -> w915
          tunnel: w914 -> [_ w934]
          frame 0, Default {
          }
          frame 75 {
            n309 = VISA Read(VISA resource name=w944, byte count=u32 3, error in (no error)=w943) -> (VISA resource name out=w939:refnum<visa-resource-name>, read buffer=w947:string, error out=w938:errorcluster)  [unwired: 1 out]
            n310 = String To Byte Array(string=w947) -> (unsigned byte array=w937:u8[])
            n311 = local read "Add Unit"() -> (w933:u8)
            n312 = Index Array(array=w937, index #1=0 ("index")) -> (element #1=w942:u8, element #2=w940:u8)  [unwired: 2 in, 1 out]
            n313 = Equal?(x=w933, y=w942) -> (x = y?=w941:bool)
            n314 = case shown="True" w941 {
              tunnel: [w954 w967] -> w950
              tunnel: [w952 w966] -> w949
              tunnel: [w951 w957] -> w948
              tunnel: w940 -> [_ w965]
              tunnel: w939 -> [w953 w964]
              tunnel: w938 -> [w952 w963]
              tunnel: w937 -> [_ w961]
              tunnel: w936 -> [w954 w958]
              tunnel: [w953 w956] -> w935
              tunnel: w934 -> [w951 w957]
              frame False {
              }
              frame True {
                n315 = VISA Read(VISA resource name=w964, byte count=w965, error in (no error)=w963) -> (VISA resource name out=w956:refnum<visa-resource-name>, read buffer=w955:string, error out=w962:errorcluster)  [unwired: 1 out]
                "RX" <- w955
                n316 = String To Byte Array(string=w955) -> (unsigned byte array=w960:u8[])
                n317 = Insert Into Array(array=w961, new element=w960) -> (w959:u8[])  [unwired: 1 in]
                n318 = Enqueue Element(queue=w958, element=w959, error in (no error)=w962) -> (queue out=w967:refnum<queue>, error out=w966:errorcluster)  [unwired: 2 out]
              }
            }
          }
        }
      }
      frame True {
        n319 = Wait (ms)(milliseconds to wait=u32 10) -> ()  [unwired: 1 out]
      }
    }
  }
  n320 = while {
    tunnel: w14 -> [_]
    tunnel: w13 -> [w974]
    stop <- "Flag Stop T" stop-if-true
    # "Transmit task"
    n321 = control-ref of="VISA"() -> (w978:refnum<vi>)
    n322 = control-ref of="CommIcon"() -> (w979:refnum<vi>)
    n323 = property class="Bool (strict)"(reference=w979) -> ("Value"=w973:bool)  [unwired: 1 in, 2 out]
    n324 = property class="VISAName"(reference=w978) -> ("Value"=w977:refnum<visa-resource-name>)  [unwired: 1 in, 2 out]
    n325 = case shown="False" w973 {
      tunnel: w977 -> [w981 _]
      tunnel: errorcluster {"status"=FALSE, "code"=0, "source"=""} -> [w980 _]
      tunnel: w974 -> [w983 _]
      frame False {
        n326 = Get Queue Status(queue=w983) -> (queue out=w982:refnum<queue>, # elements in queue=w984:i32)  [unwired: 1 in, 7 out]
        n327 = case shown="1, Default" w984 {
          tunnel: w982 -> [_ w992]
          tunnel: w981 -> [_ w991]
          tunnel: w980 -> [_ w989]
          frame 0 {
            n328 = local write "TX"(FALSE ("TX")) -> ()
          }
          frame 1, Default {
            n329 = Dequeue Element(queue=w992) -> (element=w988:u8[])  [unwired: 1 in, 4 out]
            "Write array" <- w988
            n330 = Byte Array To String(unsigned byte array=w988) -> (string=w986:string)
            "TX" <- w986
            n331 = VISA Write(VISA resource name=w991, write buffer=w986, error in (no error)=w989) -> (error out=→"err tx":errorcluster)  [unwired: 2 out]
            n332 = local write "TX"(TRUE ("TX")) -> ()
          }
        }
      }
      frame True {
        n333 = Wait (ms)(milliseconds to wait=u32 10) -> ()  [unwired: 1 out]
      }
    }
  }
